vi "connect.vi"(8 "error in (no error)":errorcluster, 11 "Electrometer in":refnum<class "Electrometer.lvclass">) -> (0 "error out":errorcluster, 2 "VISA resource name":refnum<visa-resource-name>, 3 "Electrometer out":refnum<class "Electrometer.lvclass">)   [LabVIEW 2016, in "Electrometer.lvclass"]
uses:
  Electrometer.lvclass
  <vilib>/Utility/error.llb/DialogType.ctl
  ElectrometerConfiguration.lvclass
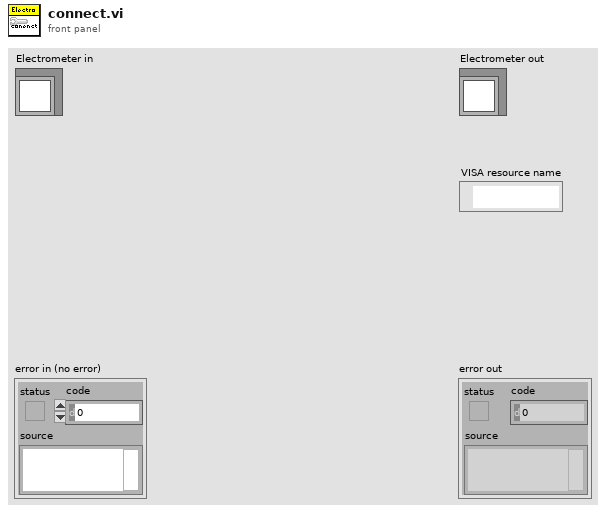
[diagram p1: front panel]
types:
  T1 = typedef "DialogType.ctl" = u16
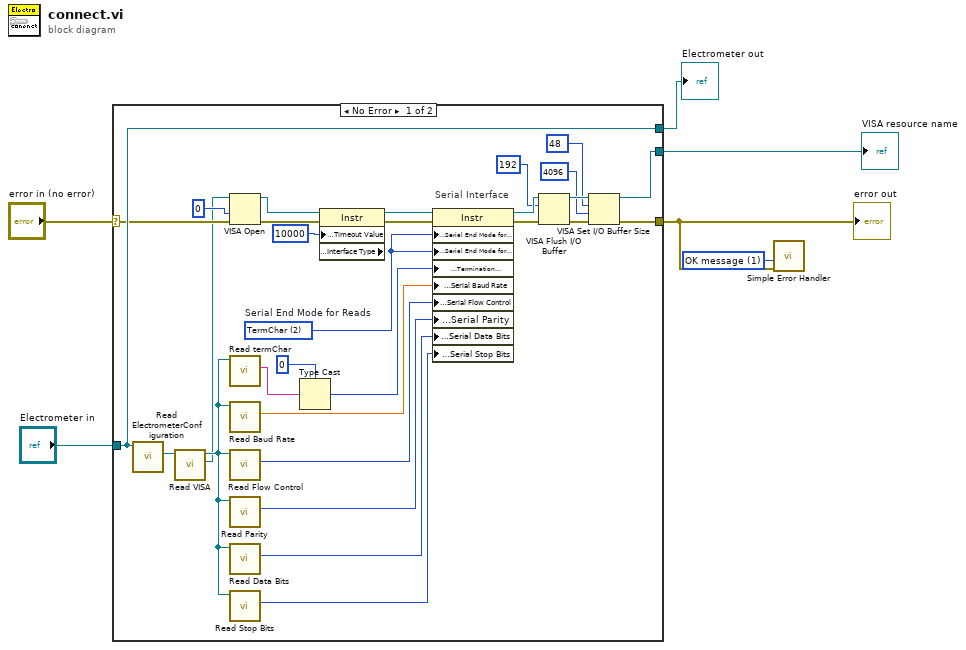
[diagram p0: block diagram]
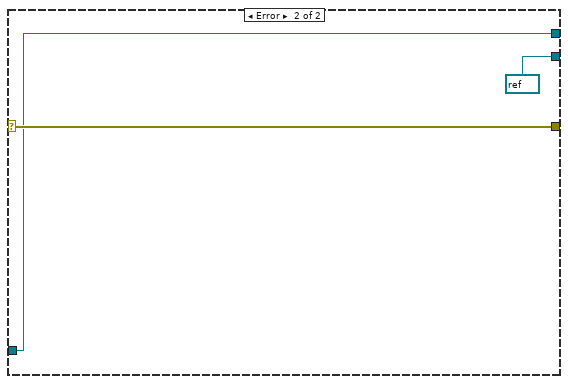
[diagram p2: hidden frame]
diagram:
  w1 = T1 1 items=["no dialog", "OK message", "continue or stop message", "OK message + warnings", "continue/stop + warnings"] ("type of dialog (OK msg:1)")
  n1 = case shown="No Error" "error in (no error)" {
    selector: "error in (no error)" -> [w12 w38]
    tunnel: [w25 w38] -> w2
    tunnel: [w24 w37] -> w4
    tunnel: "Electrometer in" -> [w24 w37]
    tunnel: [w17 refnum<visa-resource-name> refnum ("VISA resource name")] -> w3
    frame No Error {
      w27 = u16 2 items=["None", "LastBit", "TermChar"]  # Serial End Mode for Reads
      # "Serial Interface"
      n2 = call-dynamic "Read ElectrometerConfiguration.vi"("Electrometer in"=w24) -> ("ElectrometerConfiguration.lvclass"=w10:refnum<class "ElectrometerConfiguration.lvclass">)  [unwired: 8 in, 2 out]
      n3 = call-dynamic "Read VISA.vi"("ElectrometerConfiguration in"=w10) -> ("VISA"=w8:refnum<visa-resource-name>, "ElectrometerConfiguration out"=w9:refnum<class "ElectrometerConfiguration.lvclass">)  [unwired: 8 in, 1 out]
      n4 = VISA Open(access mode=u32 0, error in (no error)=w12, VISA resource name=w8) -> (VISA resource name=w14:refnum<visa-resource-name>, error out=w13:errorcluster)  [unwired: 2 in]
      n5 = call-dynamic "Read termChar.vi"("ElectrometerConfiguration in"=w9) -> ("termChar"=w18:string)  [unwired: 8 in, 2 out]
      n6 = call-dynamic "Read Baud Rate.vi"("ElectrometerConfiguration in"=w9) -> ("Baud Rate"=w20:dbl)  [unwired: 8 in, 2 out]
      n7 = call-dynamic "Read Flow Control.vi"("ElectrometerConfiguration in"=w9) -> ("Flow Control"=w21:u16)  [unwired: 8 in, 2 out]
      n8 = call-dynamic "Read Parity.vi"("ElectrometerConfiguration in"=w9) -> ("Parity"=w22:u16)  [unwired: 8 in, 2 out]
      n9 = call-dynamic "Read Data Bits.vi"("ElectrometerConfiguration in"=w9) -> ("Data Bits"=w19:u16)  [unwired: 8 in, 2 out]
      n10 = call-dynamic "Read Stop Bits.vi"("ElectrometerConfiguration in"=w9) -> ("Stop Bits"=w23:u16)  [unwired: 8 in, 2 out]
      n11 = Type Cast(type=u8 0, x=w18) -> (*(type *) &x=w26:u8)
      n12 = property class="Instr" props=["General Settings:Timeout Value", "Interface Information:Interface Type"](reference=w14, error in=w13, "General Settings:Timeout Value"=u32 10000) -> (reference out=w7:refnum<visa-resource-name>, error out=w11:errorcluster)  [unwired: 1 out]
      n13 = property class="Instr"(reference=w7, error in=w11, "Serial Settings:Serial End Mode for Reads"=w27, "Serial Settings:Serial End Mode for Writes"=w27, "Message Based Settings:Termination Character"=w26, "Serial Settings:Serial Baud Rate"=w20, "Serial Settings:Serial Flow Control"=w21, "Serial Settings:Serial Parity"=w22, "Serial Settings:Serial Data Bits"=w19, "Serial Settings:Serial Stop Bits"=w23) -> (reference out=w32:refnum<visa-resource-name>, error out=w34:errorcluster)
      n14 = VISA Flush I/O Buffer(VISA resource name=w32, mask (16)=u16 192, error in (no error)=w34) -> (VISA resource name out=w35:refnum<visa-resource-name>, error out=w33:errorcluster)
      n15 = VISA Set I/O Buffer Size(VISA resource name=w35, mask (16)=u16 48, size (4096)=u32 4096 ("size (0)"), error in (no error)=w33) -> (VISA resource name out=w17:refnum<visa-resource-name>, error out=w25:errorcluster)
    }
    frame Error {
    }
  }
  "error out" <- w2
  "Electrometer out" <- w4
  "VISA resource name" <- w3
  n16 = call <vilib>:"Simple Error Handler.vi"("type of dialog (OK msg:1)"=w1, "error in (no error)"=w2) -> ()  [unwired: 3 in, 5 out]
